vi "chirp.vi"() -> ()   [LabVIEW 2024]
uses:
  <instrlib>/niUSRP/niUSRP Write Tx Data (CDB).vi
  <vilib>/Analysis/NI_AALBase.lvlib
panel:
  out "Waveform Graph":dbl[](graph)
  in  "Chirp Patern":i32=128
  in  "EndingFrequency":dbl
  in  "SampleRate":dbl
  in  "BeginningFrequency":dbl
  in  "Amplitude":dbl=1.0 format="%0.2f"
  in  "Abort":bool
  in  "active antenna":string
  in  "gain":dbl format="%#_6f"
  in  "Carrier Frequency":dbl=100000.0 format="%#_6p"
  in  "IQ rate":dbl=100000.0 format="%#_6p"
  in  "device names":refnum<k15>
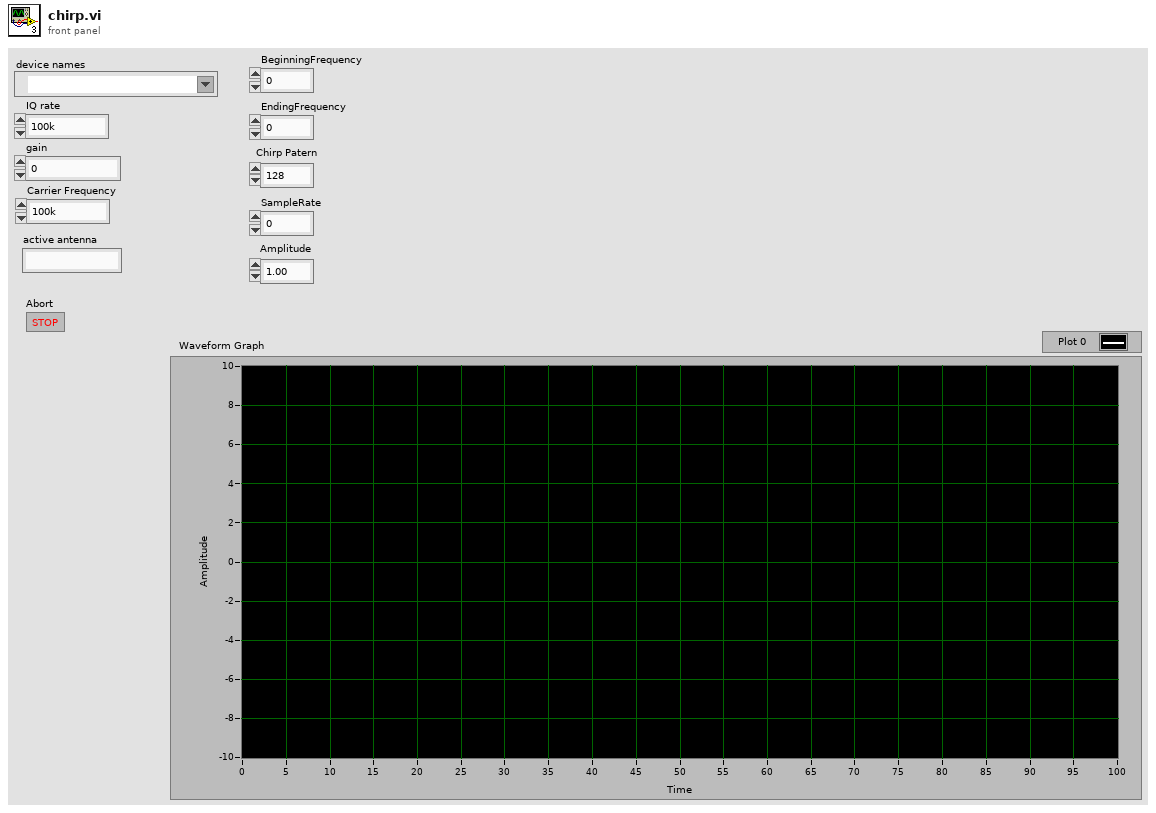
[diagram p1: front panel]
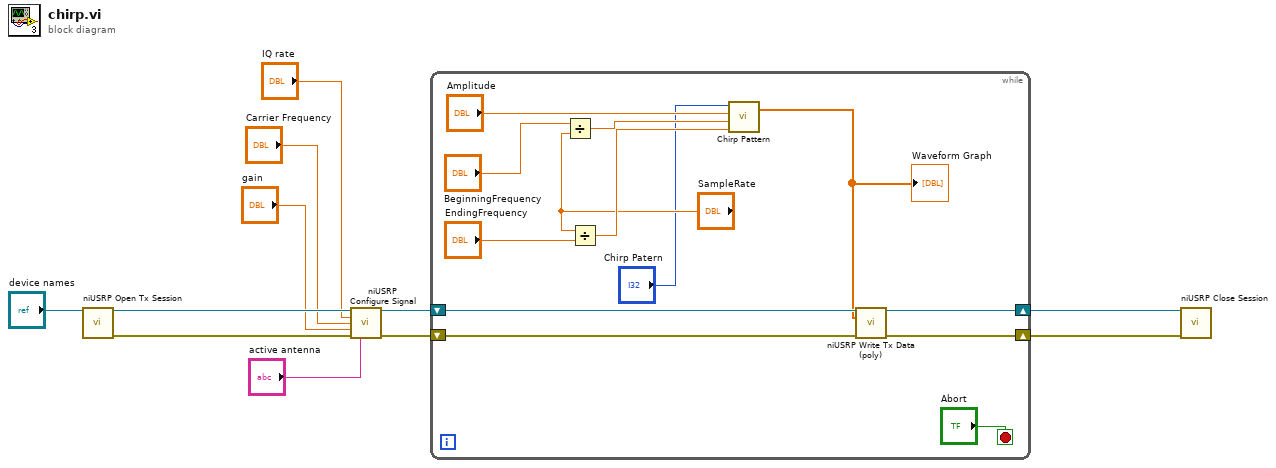
[diagram p0: block diagram]
diagram:
  n1 = call <instrlib>:"niUSRP Open Tx Session.vi"("device names"="device names") -> ("session handle out"=w10:refnum<k15>, "error out"=w9:errorcluster)  [unwired: 13 in]
  n2 = call <instrlib>:"niUSRP Configure Signal.vi"("session handle"=w10, "IQ rate"="IQ rate", "carrier frequency"="Carrier Frequency", "gain"="gain", "error in (no error)"=w9, "active antenna"="active antenna") -> ("session handle out"=w8:refnum<k15>, "error out"=w5:errorcluster)  [unwired: 5 in, 3 out]
  n3 = while {
    shift-right: [w23] -> w7
    shift-left: w8 -> [w24]
    shift-right: [w22] -> w6
    shift-left: w5 -> [w21]
    stop <- "Abort" stop-if-true
    n4 = Divide(x="BeginningFrequency", y="SampleRate") -> (x/y=w18:dbl)
    n5 = Divide(x="SampleRate", y="EndingFrequency") -> (x/y=w17:dbl)
    n6 = call <vilib>:"Chirp Pattern.vi"("f2"=w17, "f1"=w18, "amplitude"="Amplitude", "samples"="Chirp Patern") -> ("Chirp Pattern"=w12:dbl[])  [unwired: 1 out]
    "Waveform Graph" <- w12
    n7 = call-poly <instrlib>:"niUSRP Write Tx Data (poly).vi"("session handle"=w24, "data"=w12, "error in (no error)"=w21) -> ("session handle out"=w23:refnum<k15>, "error out"=w22:errorcluster)  [unwired: 11 in]
  }
  n8 = call <instrlib>:"niUSRP Close Session.vi"("session handle"=w7, "error in (no error)"=w6) -> ()  [unwired: 13 in, 1 out]
